vi "addMN.vi"(8 "error in (no error)":errorcluster caption="错误输入（无错误）", 10 "簇":cluster{"MN":string, "PW":string}={"MN"="平台数据发送系统", "PW"="平台数据发送系统"}, 11 "interface 输入":refnum<class "interface.lvclass">) -> (0 "error out":errorcluster caption="错误输出", 2 "添加成功标记":bool, 3 "interface 输出":refnum<class "interface.lvclass">)   [LabVIEW 2016, in "interface.lvclass"]
uses:
  interface.lvclass
  <vilib>/registry/registry.llb/Registry RtKey.ctl
  <vilib>/registry/registry.llb/Write Registry Value Simple STR.vi
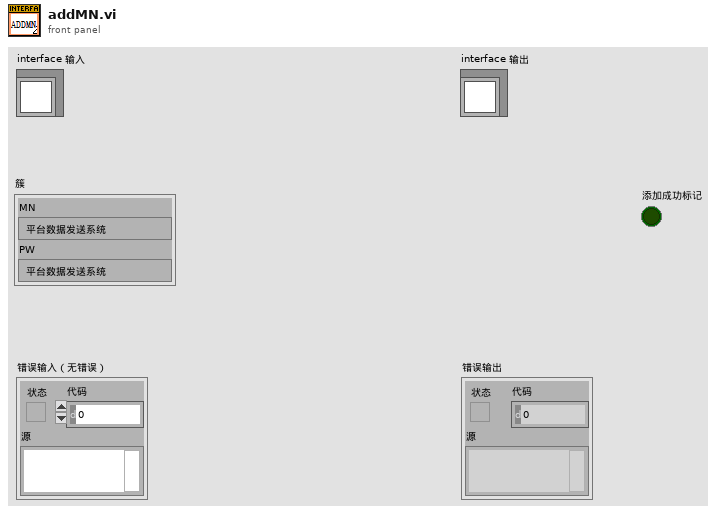
[diagram p1: front panel]
types:
  T1 = typedef "Registry RtKey.ctl" = enum32{"HKEY_CLASSES_ROOT", "HKEY_CURRENT_USER", "HKEY_LOCAL_MACHINE", "HKEY_USERS", "HKEY_PERFORMANCE_DATA", "HKEY_CURRENT_CONFIG", "HKEY_DYN_DATA"}
  T2 = typedef "Registry refnum.ctl" = refnum<k1>
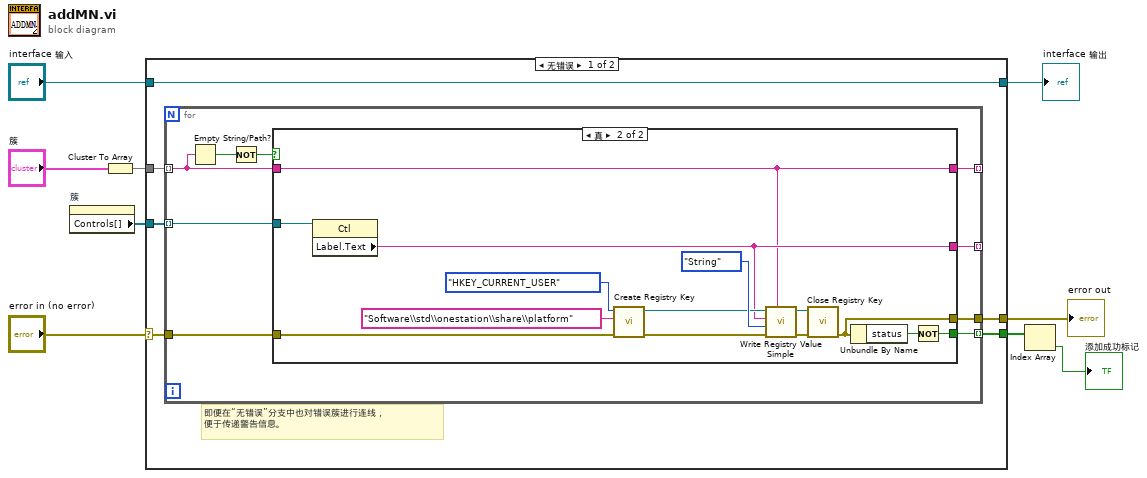
[diagram p0: block diagram]
diagram:
  n1 = property on="簇" class="Clust (严格)"() -> ("Controls[]"=w3:refnum<vi>[])  [unwired: 2 in, 2 out]
  n2 = Cluster To Array(cluster="簇") -> (array=w4:string[])
  n3 = case shown="无错误" "error in (no error)" {
    selector: "error in (no error)" -> [w10 w40]
    tunnel: [w11 w40] -> w8
    tunnel: [w15 w39] -> w6
    tunnel: "interface 输入" -> [w15 w39]
    tunnel: w4 -> [w14 _]
    tunnel: w3 -> [w13 _]
    tunnel: [w12 _] -> w1
    frame No Error {
      # "即便在“无错误”分支中也对错误簇进行连线，\n便于传递警告信息。"
      n4 = for {
        tunnel: w14 -> [w22] mode=indexing
        tunnel: w13 -> [w21] mode=indexing
        tunnel: [w20] -> _ mode=indexing
        tunnel: [w19] -> _ mode=indexing
        tunnel: [w18] -> w12 mode=indexing
        tunnel: [w17] -> w11
        tunnel: w10 -> [w16]
        n5 = Empty String/Path?(string/path=w22) -> (empty?=w24:bool)
        n6 = Not(x=w24) -> (.not. x?=w23:bool)
        n7 = case shown="真" w23 {
          tunnel: w22 -> [_ w27]
          tunnel: [_ w34] -> w18
          tunnel: w21 -> [_ w29]
          tunnel: [_ w28] -> w20
          tunnel: [_ w27] -> w19
          tunnel: [_ w26] -> w17
          tunnel: w16 -> [_ w25]
          frame False {
          }
          frame True {
            n8 = property class="Ctl"(reference=w29) -> ("Label.Text"=w28:string)  [unwired: 1 in, 2 out]
            n9 = call <vilib>:"Create Registry Key.vi"("error in (no error)"=w25, "subkey"="Software\\std\\onestation\\share\\platform", "root key (HKEY_LOCAL_MACHINE)"=Registry_RtKey."HKEY_CURRENT_USER") -> ("error out"=w30:errorcluster, "refnum out"=w31:T2)  [unwired: 6 in, 1 out]
            n10 = call-poly <vilib>:"Write Registry Value Simple.vi"("String/Binary data"=w27, "error in (no error)"=w30, "simple data type"=enum16{"String", "Binary", "DWORD"}."String", "value"=w28, "refnum"=w31) -> ("error out"=w38:errorcluster, "refnum out"=w37:T2)  [unwired: 3 in]
            n11 = call <vilib>:"Close Registry Key.vi"("error in (no error)"=w38, "refnum"=w37) -> ("error out"=w26:errorcluster)  [unwired: 5 in]
            n12 = Unbundle By Name(w26) -> ("status"=w35:bool)
            n13 = Not(x=w35) -> (.not. x?=w34:bool)
          }
        }
      }
    }
    frame Error {
    }
  }
  "error out" <- w8
  "interface 输出" <- w6
  n14 = Index Array(array=w1) -> (element=→"添加成功标记":bool)  [unwired: 1 in]
